vi "FormatIntoString.vi"() -> ()   [LabVIEW 2019]
panel:
  out "String":string
  in  "temp":dbl
  in  "b":u8
  in  "a":u8
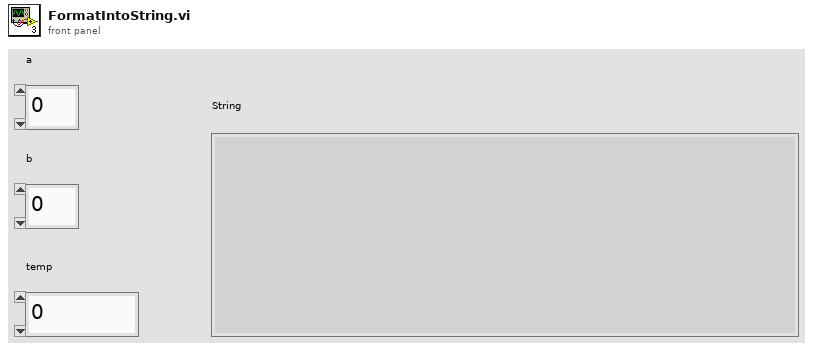
[diagram p1: front panel]
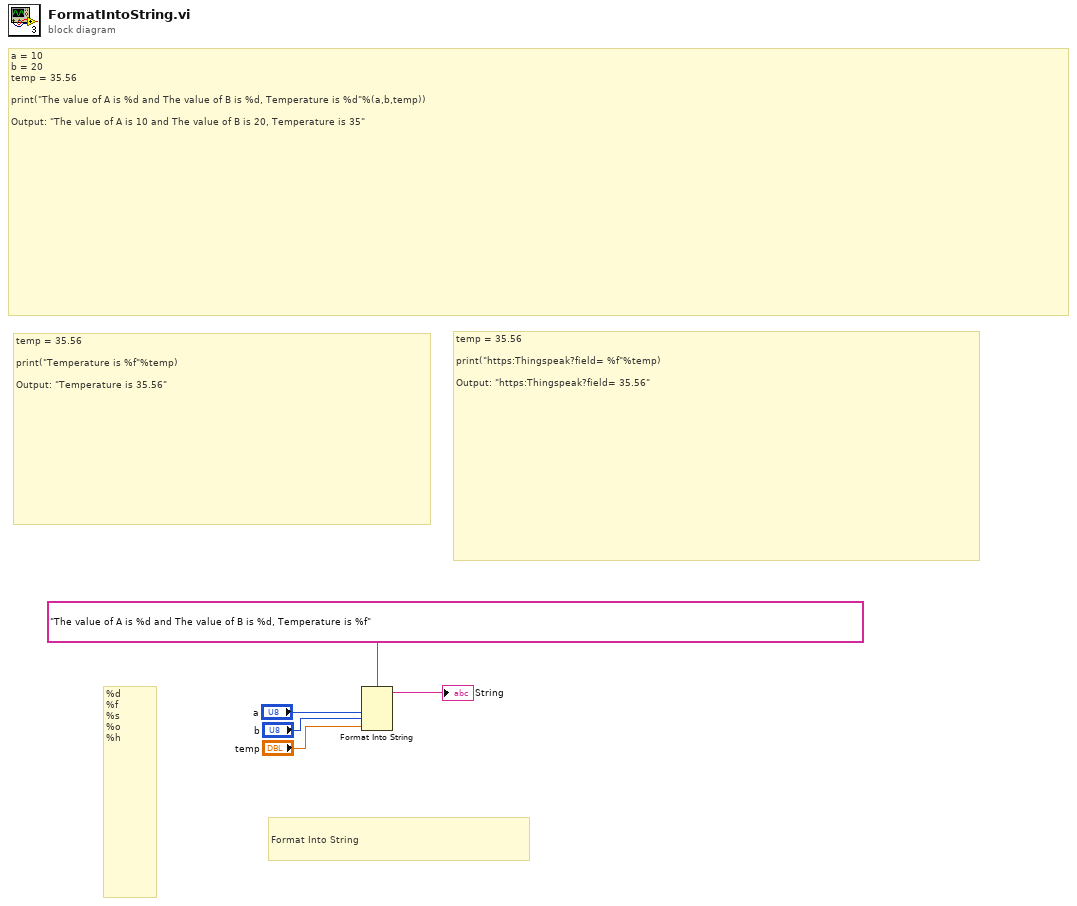
[diagram p0: block diagram]
diagram:
  # "Format Into String"
  # "%d\n%f\n%s\n%o\n%h"
  # "temp = 35.56\n\nprint(\"https:Thingspeak?field= %f\"%temp)\n\nOutput: \"https:Thingspeak?field= 35.56\""
  # "temp = 35.56\n\nprint(\"Temperature is %f\"%temp)\n\nOutput: \"Temperature is 35.56\""
  # "a = 10\nb = 20\ntemp = 35.56\n\nprint(\"The value of A is %d and The value of B is %d, Temperature is %d\"%(a,b,temp))\n\nOutput: \"The value of A is 10 and The value of B is 20, Temperature is 35\""
  n1 = Format Into String(format string="The value of A is %d and The value of B is %d, Temperature is %f", "a", "b", "temp") -> (resulting string=→"String":string)  [unwired: 2 in, 1 out]
